vi "大於0.9的時間.vi"() -> ()   [LabVIEW 2017]
panel:
  out "暫存器":bool
  out "最近十筆大於0.9":dbl[][](array[numeric])
  out "大於":bool
  out "成果陣列":dbl[][](array[numeric])
  out "小於":bool
  out "最新十筆":dbl[][](array[numeric])
  in  "迴圈速率":u32
  out "最新數據":dbl[](array[numeric])
  out "day":dbl(knob) scale=0.0..10.0
  out "hr":dbl(knob) scale=0.0..10.0
  out "min":dbl(knob) scale=0.0..60.0
  out "迴圈次數":i32
  in  "?":bool
  out "s":dbl(knob) scale=0.0..60.0
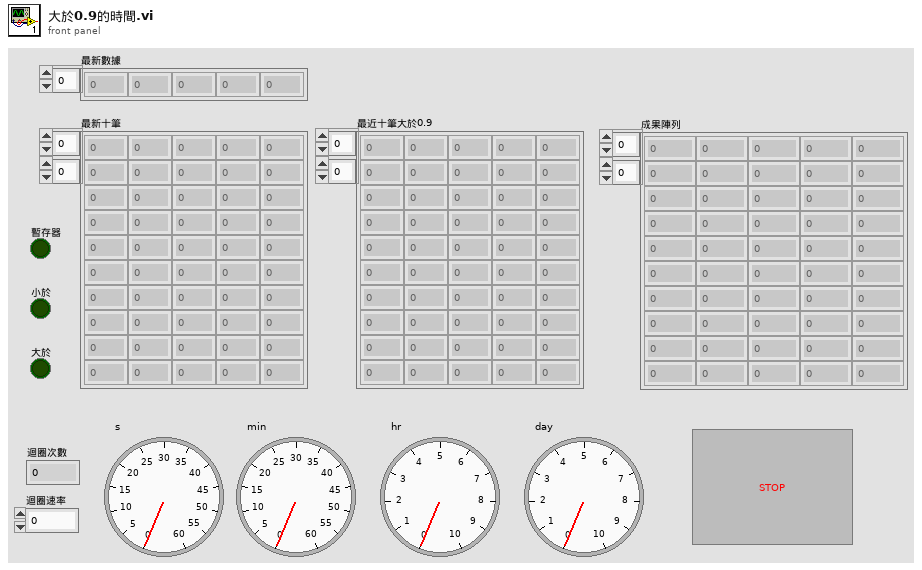
[diagram p1: front panel]
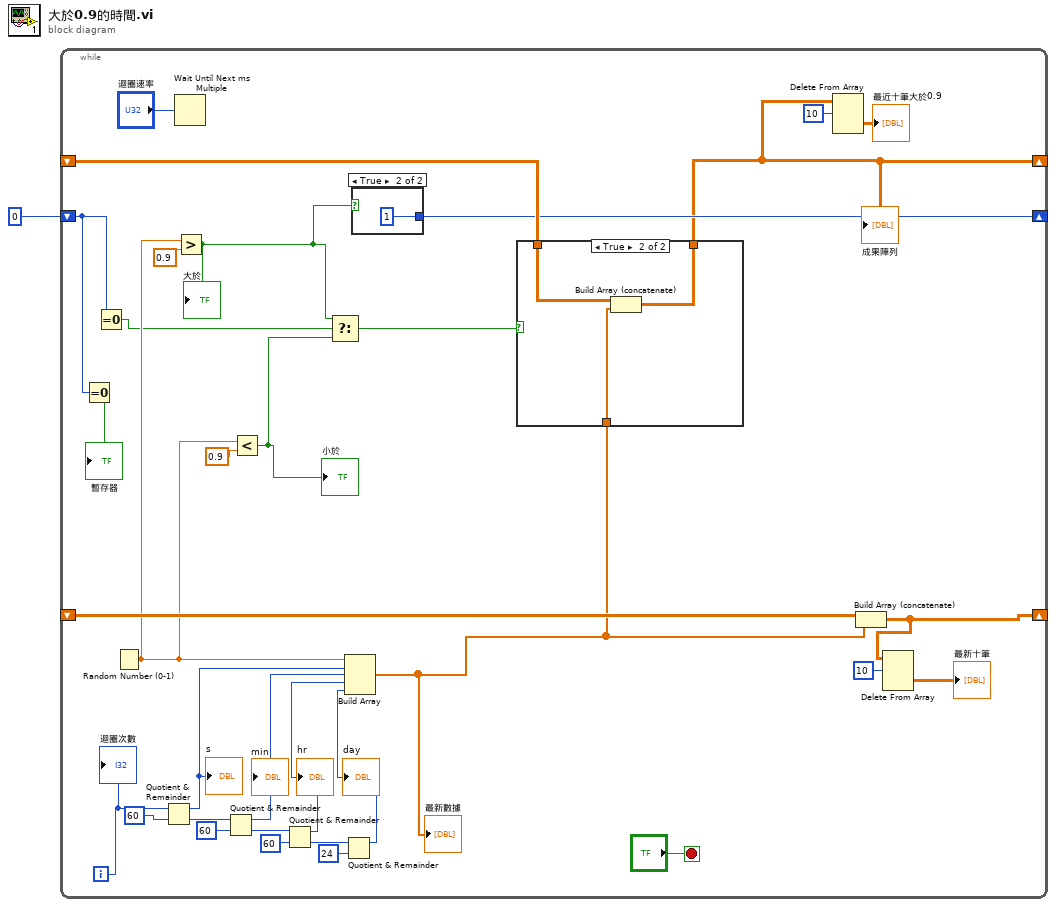
[diagram p0: block diagram]
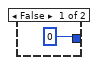
[diagram p2: hidden frame]
diagram:
  n1 = while {
    shift-right: [w18] -> _
    shift-left: _ -> [w19]
    shift-right: [w6] -> _
    shift-left: _ -> [w12]
    shift-right: [w7] -> _
    shift-left: 0 -> [w2]
    i -> [w33]
    stop <- "?" stop-if-true
    n2 = Equal To 0?(x=w2) -> (x = 0?=→"暫存器":bool)
    n3 = Equal To 0?(x=w2) -> (x = 0?=w10:bool)
    n4 = Random Number (0-1)() -> (number: 0 to 1=w14:dbl)
    n5 = Quotient & Remainder(x=w33, y=60) -> (x-y*floor(x/y)=w25:i32, floor(x/y)=w31:i32)
    "s" <- w25
    n6 = Wait Until Next ms Multiple(millisecond multiple="迴圈速率") -> ()  [unwired: 1 out]
    n7 = Greater?(x=w14, y=0.9) -> (0:w8:bool)
    "大於" <- w8
    n8 = Quotient & Remainder(x=w31, y=60) -> (x-y*floor(x/y)=w24:i32, floor(x/y)=w29:i32)
    "min" <- w24
    n9 = Less?(x=w14, y=0.9) -> (x < y?=w9:bool)
    "小於" <- w9
    n10 = Quotient & Remainder(x=w29, y=60) -> (x-y*floor(x/y)=w23:i32, floor(x/y)=w27:i32)
    "hr" <- w23
    n11 = Select(t=w8, s=w10, f=w9) -> (s? t:f=w13:bool)
    n12 = Quotient & Remainder(x=w27, y=24) -> (x-y*floor(x/y)=w22:i32)  [unwired: 1 out]
    "day" <- w22
    n13 = Build Array(w14, w25, w24, w23, w22) -> (w11:dbl[])
    "最新數據" <- w11
    n14 = case shown="True" w8 {
      tunnel: [0 1] -> w7
      frame False {
      }
      frame True {
      }
    }
    n15 = case shown="True" w13 {
      tunnel: w12 -> [w37 w40]
      tunnel: [w37 w38] -> w6
      tunnel: w11 -> [_ w39]
      frame False {
      }
      frame True {
        n16 = Build Array (concatenate)(w40, w39) -> (w38:dbl[][])
      }
    }
    "成果陣列" <- w6
    n17 = Delete From Array(array=w6, length=10) -> (deleted portion=→"最近十筆大於0.9":dbl[][])  [unwired: 2 in, 1 out]
    n18 = Build Array (concatenate)(w19, w11) -> (w18:dbl[][])
    n19 = Delete From Array(array=w18, length=10) -> (deleted portion=→"最新十筆":dbl[][])  [unwired: 2 in, 1 out]
    "迴圈次數" <- w33
  }
